vi "Update Joint Angles.vi"(8 "error in (no error)":errorcluster, 11 "GripsMaster in":refnum<class "GripsMaster.lvclass">) -> (0 "error out":errorcluster, 3 "GripsMaster out":refnum<class "GripsMaster.lvclass">)   [LabVIEW 2011, in "GripsMaster.lvclass"]
uses:
  GripsMaster.lvclass
  GripsMaster.lvclass/GripsMaster.ctl
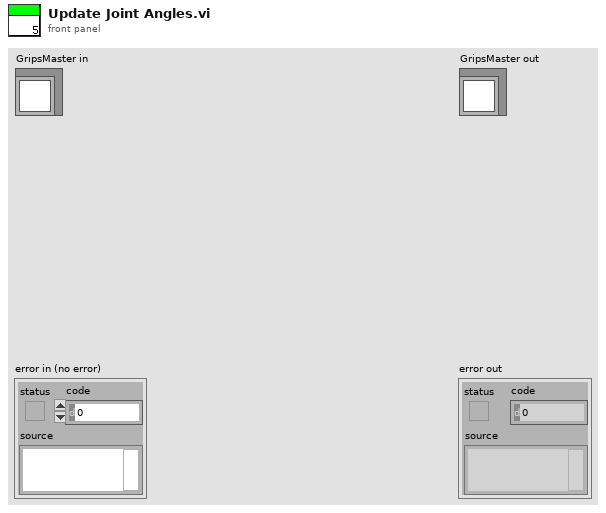
[diagram p1: front panel]
types:
  T1 = typedef "Digital Values.ctl" = cluster{"names":string[], "values":bool[]}
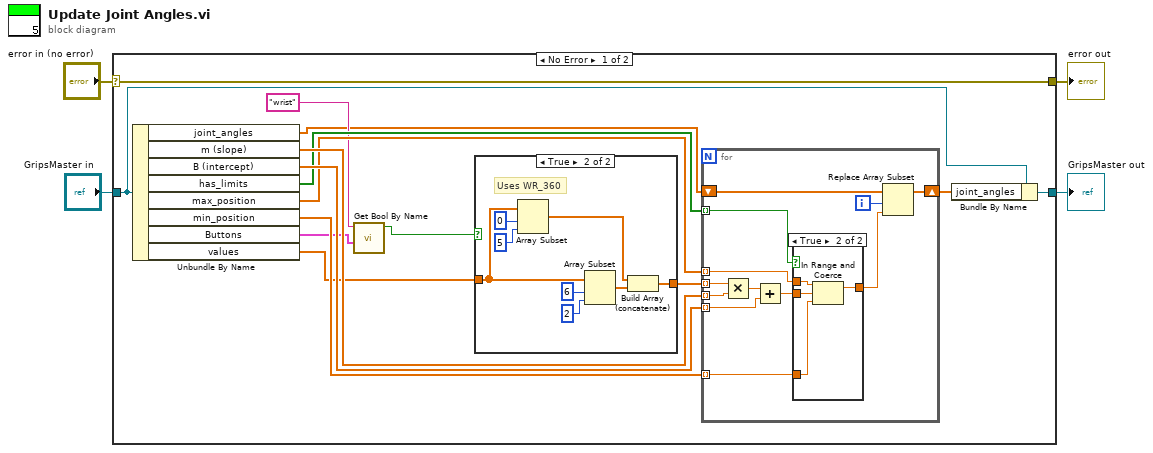
[diagram p0: block diagram]
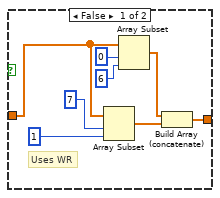
[diagram p2: hidden frame]
diagram:
  n1 = case shown="No Error" "error in (no error)" {
    selector: "error in (no error)" -> [w19 w54]
    tunnel: [w19 w54] -> w3
    tunnel: [w12 w53] -> w1
    tunnel: "GripsMaster in" -> [w13 w53]
    frame No Error {
      n2 = Unbundle By Name(w13) -> ("joint_angles"=w8:dbl[], "m (slope)"=w18:dbl[], "B (intercept)"=w17:dbl[], "has_limits"=w16:bool[], "max_position"=w15:dbl[], "min_position"=w14:dbl[], "Buttons"=w6:T1, "values"=w7:dbl[])
      n3 = call "Get Bool By Name.vi"("name"="wrist", "Digital Values"=w6) -> ("result"=w5:bool)  [unwired: 7 in, 1 out]
      n4 = case shown="True" w5 {
        tunnel: w7 -> [w22 w29]
        tunnel: [w20 w28] -> w9
        frame False {
          # "Uses WR"
          n5 = Array Subset(array=w22, index=7, length=1) -> (w23:dbl[])
          n6 = Array Subset(array=w22, index=0, length=6) -> (w24:dbl[])
          n7 = Build Array (concatenate)(w24, w23) -> (w20:dbl[])
        }
        frame True {
          # "Uses WR_360"
          n8 = Array Subset(array=w29, index=0, length=5) -> (w31:dbl[])
          n9 = Array Subset(array=w29, index=6, length=2) -> (w30:dbl[])
          n10 = Build Array (concatenate)(w31, w30) -> (w28:dbl[])
        }
      }
      n11 = for {
        tunnel: w18 -> [w46] mode=indexing
        tunnel: w17 -> [w44] mode=indexing
        tunnel: w9 -> [w47] mode=indexing
        tunnel: w16 -> [w43] mode=indexing
        tunnel: w15 -> [w41] mode=indexing
        tunnel: w14 -> [w40] mode=indexing
        shift-right: [w36] -> w11
        shift-left: w8 -> [w38]
        i -> [w39]
        n12 = Multiply(x=w47, y=w46) -> (x*y=w45:dbl)
        n13 = Add(x=w45, y=w44) -> (x+y=w42:dbl)
        n14 = case shown="True" w43 {
          tunnel: w42 -> [w48 w52]
          tunnel: w41 -> [_ w51]
          tunnel: w40 -> [_ w50]
          tunnel: [w48 w49] -> w37
          frame False {
          }
          frame True {
            n15 = In Range and Coerce(upper limit=w51, x=w52, lower limit=w50) -> (coerced(x)=w49:dbl)  [unwired: 1 out]
          }
        }
        n16 = Replace Array Subset(array=w38, new element=w37, index=w39) -> (w36:dbl[])
      }
      n17 = Bundle By Name(cluster=w13, "joint_angles"=w11) -> (w12:refnum<class "GripsMaster.lvclass">)
    }
    frame Error {
    }
  }
  "error out" <- w3
  "GripsMaster out" <- w1
